vi "mqtt_data_test.vi"() -> ()   [LabVIEW 2019]
uses:
  src/class/mqtt/mqttTypedef/mqttConnectionStatus.ctl
  src/class/mqtt/mqttTypedef/mqttSubscribeCluster.ctl
  src/class/mqtt/mqttTypedef/mqttQOSlevel.ctl
  src/class/mqtt/mqttTypedef/mqttBroker.ctl
  src/class/mqtt/mqttTypedef/mqttConnectionFlags.ctl
  src/class/mqtt/mqttTypedef/mqttWillInformation.ctl
  src/class/mqtt/mqttConfigFunction.ctl
  src/class/mqtt/mqttTXqueue/mqttTXdataQueueFunction.ctl
  src/class/mqtt/mqttTXqueue/mqttRXsubscriptionEventFunction.ctl
  src/class/mqtt/mqtt.lvclass
panel:
  out "subscribeMessageID":u16 format="%02x"
  out "subscribeSuccess":bool
  in  "subscriptionInfo":T1[](array[typedef])=[{"Topic"="a/b", "QoS"=enum."At most once"}]
  out "RX Value":string
  out "RX Topic":string
  in  "subscribe":bool
  in  "topic":string
  in  "Boolean":bool
  out "x+1":i32
  out "decimal integer string":string
  in  "Slide":dbl(slide) min=0.0 max=40.0 step=0.01 scale=0.0..40.0
  out "error out":errorcluster
  in  "connect":bool
  in  "quit":bool
  in  "publish":bool
  out "sessionPresent":bool
  out "connStatus":T3=enum."Connection refused: not authorized"
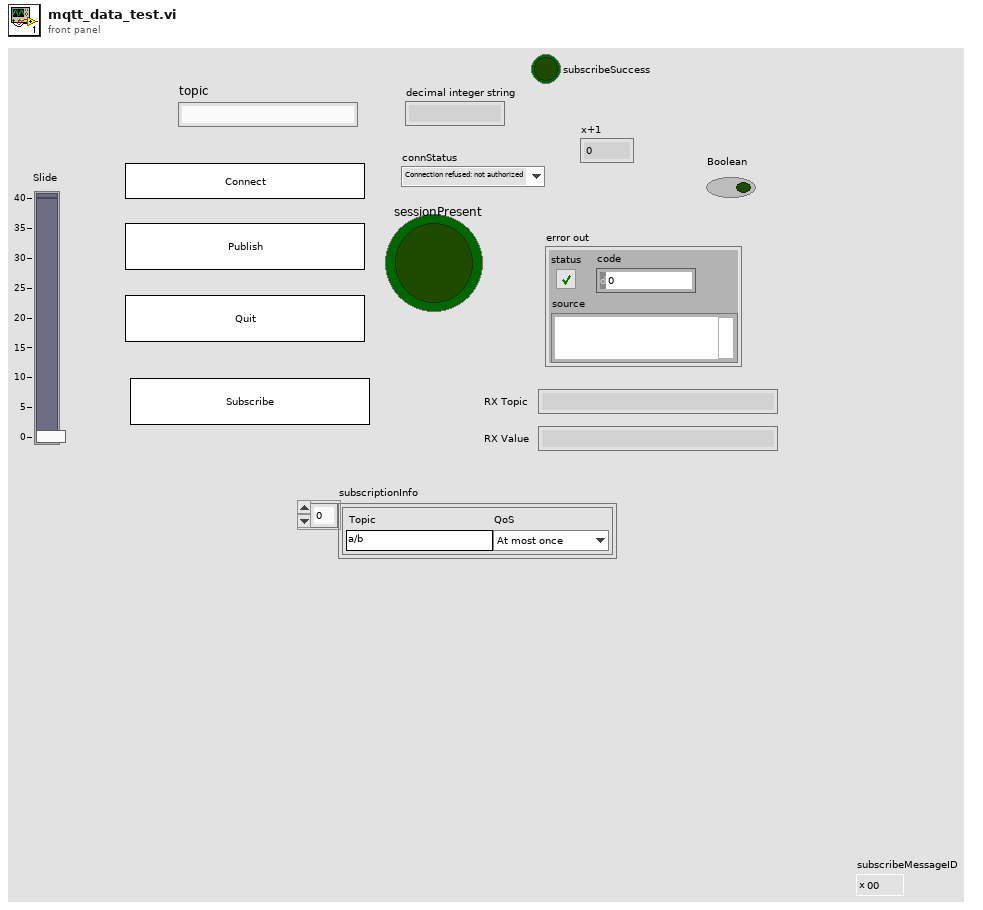
[diagram p1: front panel]
types:
  T1 = typedef "mqttSubscribeCluster.ctl" = cluster{"Topic":string, "QoS":T2}
  T2 = typedef "mqttQOSlevel.ctl" = enum8{"At most once", "At least once", "Exactly once", "Reserved"}
  T3 = typedef "mqttConnectionStatus.ctl" = enum16{"Connection accepted", "Connection refused: unacceptable protocol version", "Connection refused: identifier rejected", "Connection refused: Server unavailable", "Connection refused: bad user name or password", "Connection refused: not authorized"}
  T4 = typedef "mqttRXsubscriptionEventFunction.ctl" = enum16{"init", "deinit", "getEventRef", "event"}
  T5 = typedef "mqttTXdataQueueFunction.ctl" = enum16{"init", "deinit", "getQueue", "enqueue"}
  T6 = typedef "mqtt.lvclass/mqttConfigFunction.ctl" = enum16{"init", "deinit", "set", "get"}
  T7 = typedef "mqttWillInformation.ctl" = cluster{"User Name":string, "Password":string}
  T8 = typedef "mqttConnectionFlags.ctl" = cluster{"reserved":bool, "clean session":bool, "will flag":bool, "willQOS":enum8{"At most once", "At least once", "Exactly once", "Reserved"}, "will retain":bool, "password":bool, "user name":bool}
  T9 = typedef "mqttBroker.ctl" = cluster{"address":string, "port":u16, "connTimeout":i32, "writeTimeout":i32, "readTimeout":i32, "subTimeout":i32}
  T10 = enum8{"Enabled", "Disabled", "Disabled and Grayed Out"}
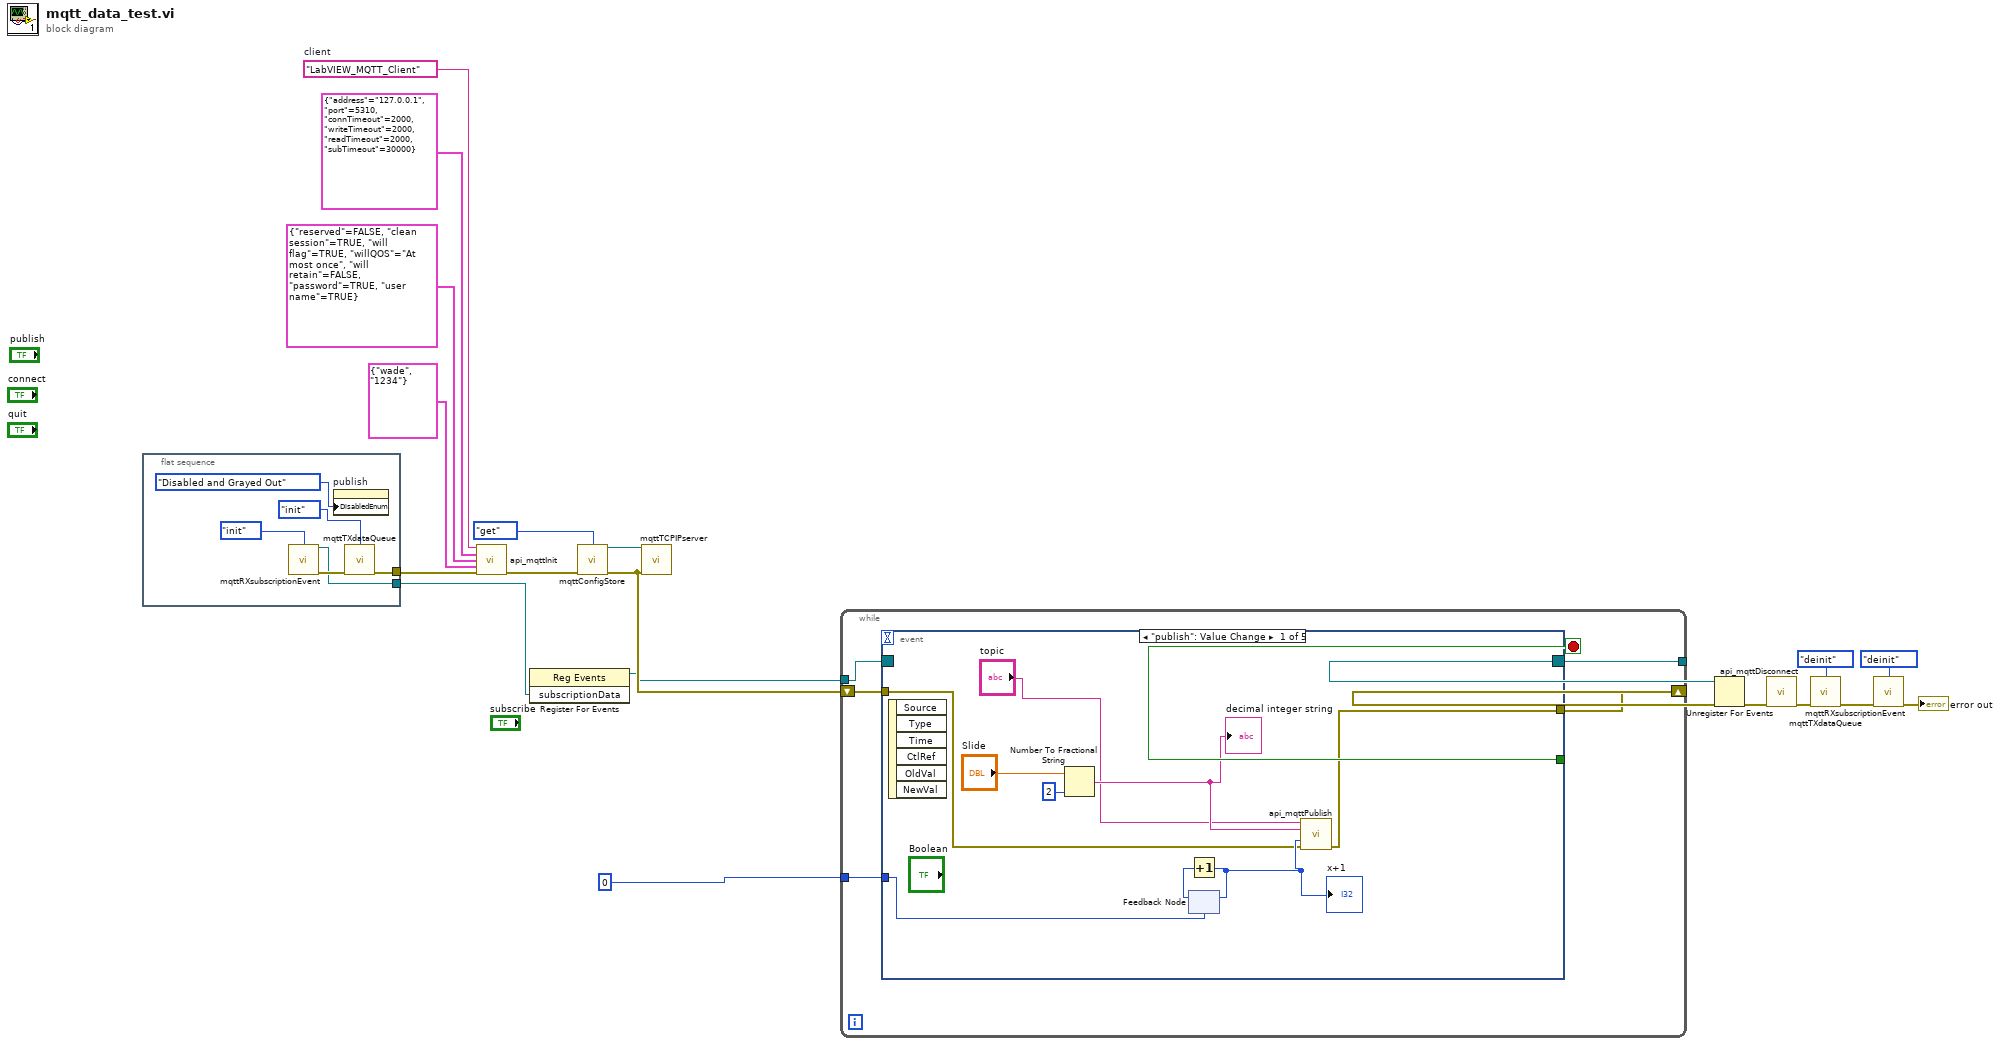
[diagram p0: block diagram]
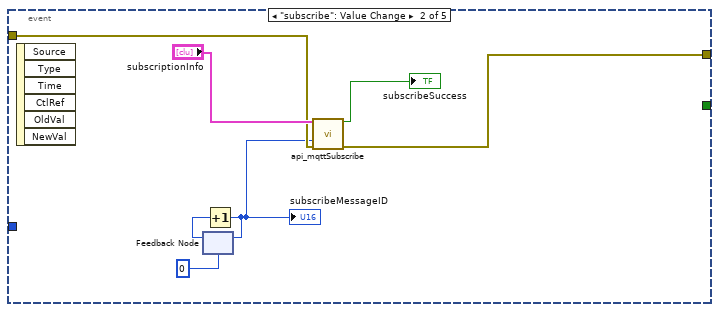
[diagram p2: hidden frame]
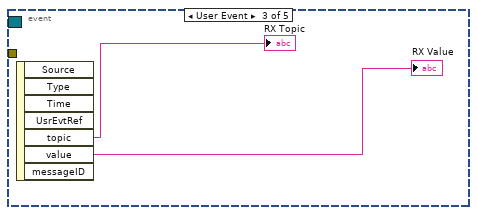
[diagram p3: hidden frame]
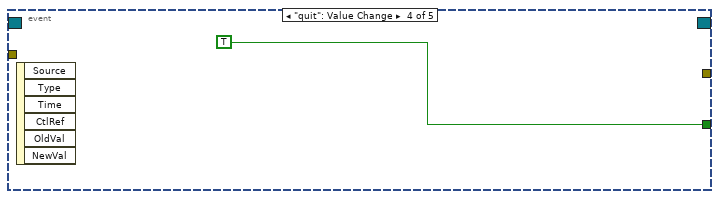
[diagram p4: hidden frame]
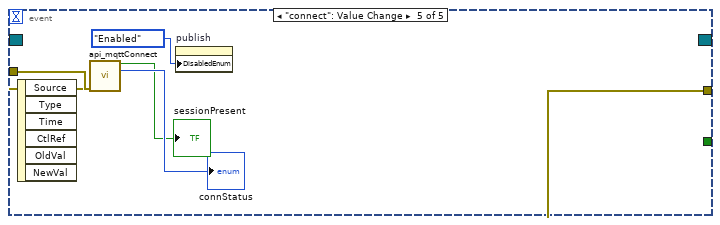
[diagram p5: hidden frame]
diagram:
  w17 = "LabVIEW_MQTT_Client"  # client
  n1 = flat-sequence {
    tunnel: [w25] -> w19
    tunnel: [w22] -> w11
    frame #0 {
      n2 = call "mqttRXsubscriptionEvent.vi"("function"=mqttRXsubscriptionEventFunction."init") -> ("subscriptionData"=w22:refnum<user-event>, "error out"=w24:errorcluster)  [unwired: 13 in]
      n3 = property on="publish" class="Bool"("DisabledEnum"=T10."Disabled and Grayed Out" ("Disabled")) -> ()  [unwired: 2 in, 2 out]
      n4 = call "mqttTXdataQueue.vi"("function"=mqttTXdataQueueFunction."init", "error in (no error)"=w24) -> ("error out"=w25:errorcluster)  [unwired: 12 in, 1 out]
    }
  }
  n5 = call "api_mqttInit.vi"("client"=w17, "broker"=T9 {"address"="127.0.0.1", "port"=5310, "connTimeout"=2000, "writeTimeout"=2000, "readTimeout"=2000, "subTimeout"=30000}, "connFlags"=T8 {"reserved"=FALSE, "clean session"=TRUE, "will flag"=TRUE, "willQOS"=enum."At most once", "will retain"=FALSE, "password"=TRUE, "user name"=TRUE}, "User Info"=T7 {"User Name"="wade", "Password"="1234"}, "error in (no error)"=w19) -> ("error out"=w18:errorcluster)  [unwired: 10 in]
  n6 = register-events(w11) -> (reference out=w10:refnum<event-registration>)  [unwired: 2 in, 1 out]
  n7 = call "mqttConfigStore.vi"("function"=mqttConfigFunction."get", "error in (no error)"=w18) -> ("mqtt.lvclass out"=w12:refnum<class "mqtt.lvclass">, "error out"=w13:errorcluster)  [unwired: 12 in]
  n8 = call "mqttTCPIPserver.vi"("mqtt.lvclass"=w12, "error in (no error)"=w13) -> ()  [unwired: 12 in, 2 out]
  n9 = while {
    tunnel: w10 -> [w29]
    shift-right: [w30] -> w3
    shift-left: w13 -> [w31]
    tunnel: [w28] -> w2
    tunnel: 0 -> [w27]
    stop <- w32 stop-if-true
    n10 = event shown="[0] \"publish\": Value Change" {
      selector: w29 -> [_ _ _ _ _]
      dyn-events: [_ _ _ _ _] -> w28
      timeout: _ -> [_ _ _ _ _]
      tunnel: [_ _ _ TRUE _] -> w32
      tunnel: w31 -> [w35 w46 _ _ w55]
      tunnel: [w34 w45 _ _ w54] -> w30
      tunnel: w27 -> [w38 _ _ _ _]
      event "publish": Value Change {
        n11 = event-data() -> ()  [unwired: 1 in, 6 out]
        n12 = Number To Fractional String(number="Slide", precision (6)=i16 2) -> (F-format string=w39:string)  [unwired: 2 in]
        "decimal integer string" <- w39
        n13 = feedback #1(w38) -> (w37:i32)
        n14 = Increment(x=w37) -> (x+1=w36:i32)
        "x+1" <- w36
        n15 = feedback-in #1(w36) -> ()
        n16 = call "api_mqttPublish.vi"("topic"="topic", "value"=w39, "messageID"=w36, "error in (no error)"=w35) -> ("error out"=w34:errorcluster)  [unwired: 10 in, 1 out]
      }
      event "subscribe": Value Change {
        n17 = event-data() -> ()  [unwired: 1 in, 6 out]
        n18 = feedback #2(u16 0) -> (w43:u16)
        n19 = Increment(x=w43) -> (x+1=w42:u16)
        "subscribeMessageID" <- w42
        n20 = feedback-in #2(w42) -> ()
        n21 = call "api_mqttSubscribe.vi"("subscriptionInfo"="subscriptionInfo", "messageID"=w42, "error in (no error)"=w46) -> ("success"=→"subscribeSuccess":bool, "error out"=w45:errorcluster)  [unwired: 11 in]
      }
      event User Event {
        n22 = event-data() -> ("topic"=→"RX Topic":string, "value"=→"RX Value":string)  [unwired: 1 in, 5 out]
      }
      event "quit": Value Change {
        n23 = event-data() -> ()  [unwired: 1 in, 6 out]
      }
      event "connect": Value Change {
        n24 = event-data() -> ()  [unwired: 1 in, 6 out]
        n25 = call "api_mqttConnect.vi"("error in (no error)"=w55) -> ("success"=→"sessionPresent":bool, "connStatus"=→"connStatus":T3, "error out"=w54:errorcluster)  [unwired: 11 in, 1 out]
        n26 = property on="publish" class="Bool"("DisabledEnum"=T10."Enabled" ("Disabled")) -> ()  [unwired: 2 in, 2 out]
      }
    }
  }
  n27 = Unregister For Events(event registration refnum=w2, error in=w3) -> (error out=w4:errorcluster)
  n28 = call "api_mqttDisconnect.vi"("error in (no error)"=w4) -> ("error out"=w8:errorcluster)  [unwired: 13 in, 1 out]
  n29 = call "mqttTXdataQueue.vi"("function"=mqttTXdataQueueFunction."deinit", "error in (no error)"=w8) -> ("error out"=w6:errorcluster)  [unwired: 12 in, 1 out]
  n30 = call "mqttRXsubscriptionEvent.vi"("function"=mqttRXsubscriptionEventFunction."deinit", "error in (no error)"=w6) -> ("error out"=→"error out":errorcluster)  [unwired: 12 in, 1 out]
